vi "Display Client Creation Status.vi"(8 "error in":errorcluster, 9 "client names":string[](array[string]), 10 "status":string[](array[string]), 11 "statusListbox in":refnum<vi>) -> (0 "error out":errorcluster, 2 "all success?":bool, 3 "statusListbox out":refnum<vi>)   [LabVIEW 2021, in "MeasurementClient Editor.lvlib"]
uses:
  MeasurementClient Editor.lvlib
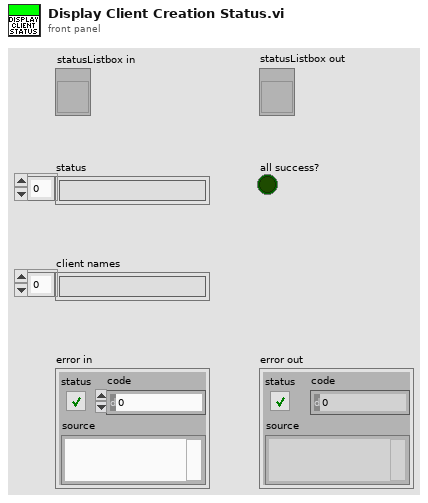
[diagram p1: front panel]
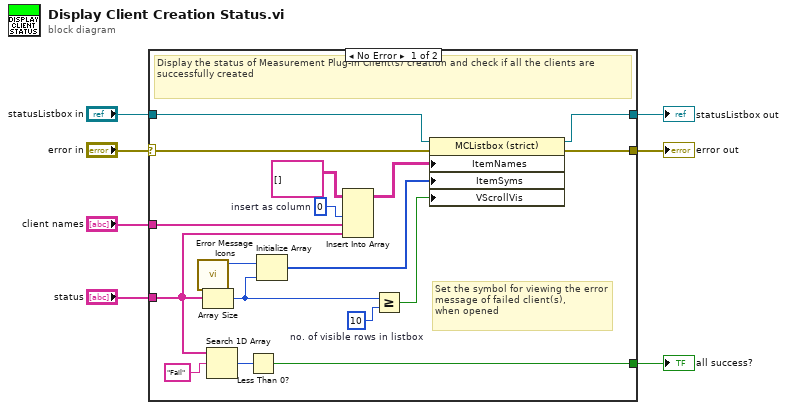
[diagram p0: block diagram]
diagram:
  n1 = case shown="No Error" "error in" {
    selector: "error in" -> [w21 w26]
    tunnel: [w23 _] -> w7
    tunnel: "statusListbox in" -> [w20 w25]
    tunnel: "client names" -> [w17 _]
    tunnel: "status" -> [w14 _]
    tunnel: [w13 w26] -> w2
    tunnel: [w12 w25] -> w1
    frame No Error {
      w9 = 10  # no. of visible rows in listbox
      w18 = 0  # insert as column
      # "Set the symbol for viewing the error message of failed client(s),\nwhen opened"
      # "Display the status of Measurement Plug-In Client(s) creation and check if all the clients are successfully created"
      n2 = call "Error Message Icons.vi"() -> ("closed"=w11:i32)  [unwired: 10 in, 1 out]
      n3 = Array Size(array=w14) -> (size(s)=w10:i32)
      n4 = Search 1D Array(1D array=w14, element="Fail") -> (index of element=w22:i32)  [unwired: 1 in]
      n5 = Less Than 0?(x=w22) -> (x < 0?=w23:bool)
      n6 = Initialize Array(w11, w10) -> (w15:i32[])
      n7 = Insert Into Array(array=string[][] [], index (col)=w18, new element #1=w17, new element #2=w14) -> (w16:string[][])  [unwired: 1 in]
      n8 = Greater Or Equal?(x=w10, y=w9) -> (x >= y?=w8:bool)
      n9 = property on="Property Node" class="MCListbox (strict)"(reference=w20, error in=w21, "ItemNames"=w16, "ItemSyms"=w15, "VScrollVis"=w8) -> (reference out=w12:refnum<vi>, error out=w13:errorcluster)
    }
    frame Error {
      # "Pass"
    }
  }
  "all success?" <- w7
  "error out" <- w2
  "statusListbox out" <- w1
